vi "niRFUtil MEAS Mean (complex wfm).vi"(7 "Waveform In":T1 {"y" format="%.2f"; "dx" format="%^.2e"; "x0" format="%^.2e"}) -> (8 "Mean":csg format="%.2f")   [LabVIEW 2015, in "niRFUtil.lvlib"]
doc: "(c) Copyright 2006, National Instruments, Inc. This VI may not be duplicated, sold, or distributed without written consent from National Instruments."
uses:
  niRFUtil.lvlib
  Includes/niRFUtil INC Complex Waveform.ctl
  Includes/niRFUtil INC Complex Array.ctl
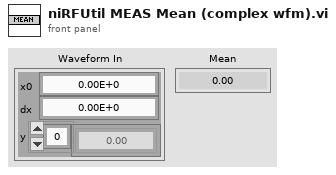
[diagram p1: front panel]
types:
  T1 = typedef "niRFUtil.lvlib/niRFUtil INC Complex Waveform.ctl" = cluster{"x0":dbl, "dx":dbl, "y":T2}
  T2 = typedef "niRFUtil.lvlib/niRFUtil INC Complex Array.ctl" = csg[]
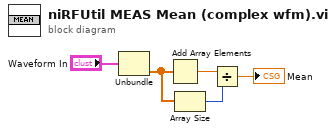
[diagram p0: block diagram]
diagram:
  n1 = Unbundle("Waveform In") -> ("y"=w2:T2)  [unwired: 2 out]
  n2 = Add Array Elements(numeric array=w2) -> (sum=w4:csg)
  n3 = Array Size(array=w2) -> (size(s)=w3:i32)
  n4 = Divide(x=w4, y=w3) -> (x/y=→"Mean":csg)
